vi "Get Arc Detect.vi"(8 "error in (no error)":errorcluster, 11 "VISA resource name":refnum<visa-resource-name>) -> (0 "error out":errorcluster, 2 "Arc Detect":bool, 3 "VISA resource name out":refnum<visa-resource-name>)   [LabVIEW 2020, in "Associated Research 78XX Series.lvlib"]
uses:
  <instrlib>/Associated Research 78XX Series/Associated Research 78XX Series.lvlib
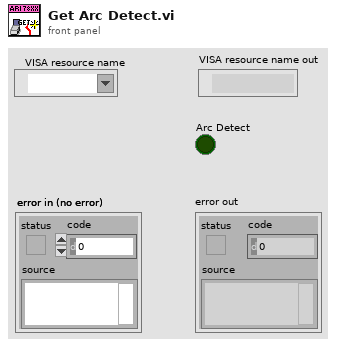
[diagram p1: front panel]
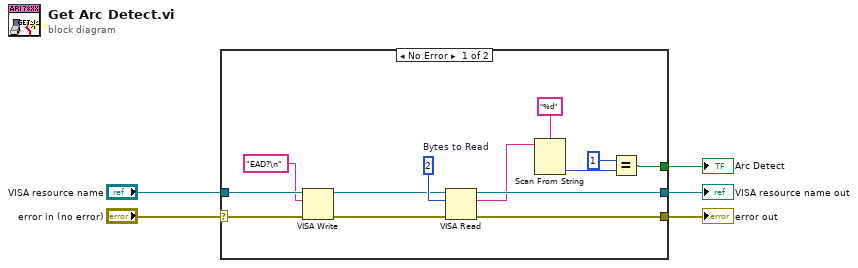
[diagram p0: block diagram]
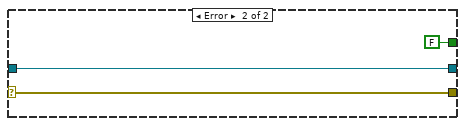
[diagram p2: hidden frame]
diagram:
  n1 = case shown="No Error" "error in (no error)" {
    selector: "error in (no error)" -> [w18 w21]
    tunnel: [w14 w21] -> w4
    tunnel: [w10 w20] -> w2
    tunnel: "VISA resource name" -> [w17 w20]
    tunnel: [w8 FALSE] -> w1
    frame No Error {
      w16 = u32 2  # Bytes to Read
      n2 = VISA Write(VISA resource name=w17, write buffer="EAD?\n" ("string (\"\")"), error in (no error)=w18) -> (VISA resource name out=w13:refnum<visa-resource-name>, error out=w12:errorcluster)  [unwired: 1 out]
      n3 = VISA Read(VISA resource name=w13, byte count=w16, error in (no error)=w12) -> (VISA resource name out=w10:refnum<visa-resource-name>, read buffer=w9:string, error out=w14:errorcluster)  [unwired: 1 out]
      n4 = Scan From String(format string="%d", input string=w9) -> (output 1=w7:i32)  [unwired: 3 in, 3 out]
      n5 = Equal?(x=1, y=w7) -> (x = y?=w8:bool)
    }
    frame Error {
    }
  }
  "error out" <- w4
  "VISA resource name out" <- w2
  "Arc Detect" <- w1
